vi "Create Image Manualy.vi"() -> ()   [LabVIEW 2017]
panel:
  out "Image":T1(plugin-control)
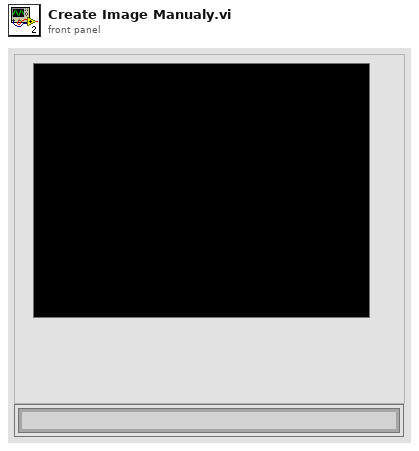
[diagram p1: front panel]
types:
  T1 = typedef "IMAQ Image.ctl" = refnum<image>
  T2 = typedef "Image Type" = u32
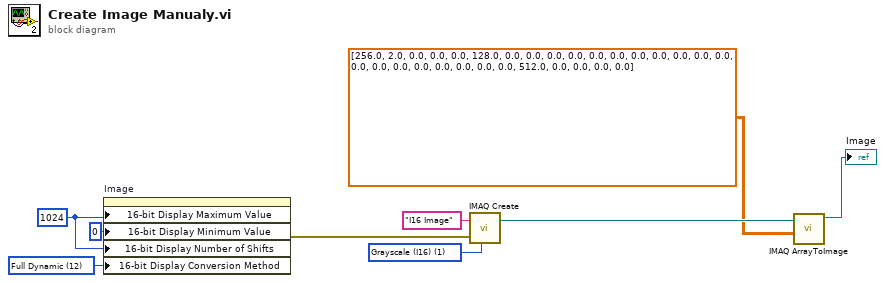
[diagram p0: block diagram]
diagram:
  w2 = u32 12 items=["Default"=10, "Most Significant Bits"=11, "Full Dynamic"=12, "Downshift"=13, "Given Range"=14, "90% Dynamic"=15, "Given Percent Range"=16] ("16-bit Display Mapping:Conversion Method")
  w3 = 1024 ("16-bit Display Mapping:Maximum Value")
  w8 = T2 1 items=["Grayscale (U8)", "Grayscale (I16)", "Grayscale (SGL)", "Complex (CSG)", "RGB (U32)", "HSL (U32)", "RGB (U64)"] ("Image Type")
  n1 = property on="Image" class="ImageControl"("16-bit Display Maximum Value"=w3, "16-bit Display Minimum Value"=0 ("16-bit Display Mapping:Minimum Value"), "16-bit Display Number of Shifts"=w3, "16-bit Display Conversion Method"=w2) -> (error out=w5:errorcluster)  [unwired: 2 in, 1 out]
  n2 = call "IMAQ Create"("Image Name"="I16 Image", "Image Type"=w8, "error in (no error)"=w5) -> ("New Image"=w6:T1)  [unwired: 2 in, 1 out]
  n3 = call "IMAQ ArrayToImage"("Image Pixels (I16)"=dbl[][] [[256.0, 2.0, 0.0, 0.0, 0.0], [128.0, 0.0, 0.0, 0.0, 0.0], [0.0, 0.0, 0.0, 0.0, 0.0], [0.0, 0.0, 0.0, 0.0, 0.0], [0.0, 0.0, 0.0, 0.0, 0.0], [512.0, 0.0, 0.0, 0.0, 0.0]], "Image"=w6) -> ("Image Out"=→"Image":T1)  [unwired: 8 in, 1 out]
